vi "NumberAverages.vi"(0 "Number in":string, 1 "String in":string) -> (7 "String out":string, 8 "Number out":string)   [LabVIEW 2015]
panel:
  in  "Counter":i32
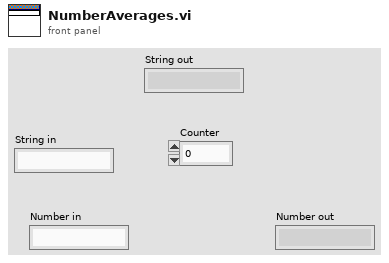
[diagram p1: front panel]
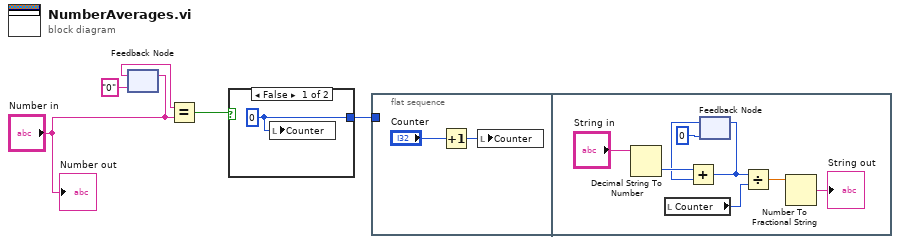
[diagram p0: block diagram]
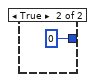
[diagram p2: hidden frame]
diagram:
  n1 = feedback #1("0" ("Number in")) -> (w3:string)
  n2 = feedback-in #1("Number in") -> ()
  n3 = Equal?(x=w3, y="Number in") -> (x = y?=w1:bool)
  n4 = case shown="False" w1 {
    tunnel: [w6 0 ("Counter")] -> w5
    frame False {
      w6 = 0 ("Counter")
      n5 = local write "Counter"(w6) -> ()
    }
    frame True {
    }
  }
  n6 = flat-sequence {
    tunnel: w5 -> [_]
    frame #0 {
      n7 = Increment(x="Counter") -> (x+1=w9:i32)
      n8 = local write "Counter"(w9) -> ()
    }
    frame #1 {
      n9 = Decimal String To Number(string="String in") -> (number=w13:i32)  [unwired: 2 in, 1 out]
      n10 = local read "Counter"() -> (w17:i32)
      n11 = feedback #2(0) -> (w11:i32)
      n12 = Add(x=w13, y=w11) -> (x+y=w12:i32)
      n13 = feedback-in #2(w12) -> ()
      n14 = Divide(x=w12, y=w17) -> (x/y=w15:dbl)
      n15 = Number To Fractional String(number=w15) -> (F-format string=→"String out":string)  [unwired: 3 in]
    }
  }
  "Number out" <- "Number in"
